vi "Set Message.vi"(8 "error in (no error)":errorcluster caption="entrée d'erreur (pas d'erreur)", 9 "Message type":T1="Control", 10 "Message.lvclass":refnum<class "Message.lvclass">, 11 "GeneralFunctionality en entrée":refnum<class "GeneralFunctionality.lvclass">) -> (0 "error out":errorcluster caption="sortie d'erreur", 3 "GeneralFunctionality en sortie":refnum<class "GeneralFunctionality.lvclass">)   [LabVIEW 2018, in "GeneralFunctionality.lvclass"]
uses:
  GeneralFunctionality.lvclass
  dependecies/ControlsVIs/Clusters-def/Message types.ctl
  Message/Message.lvclass
  GeneralFunctionality.lvclass/GeneralFunctionality.ctl
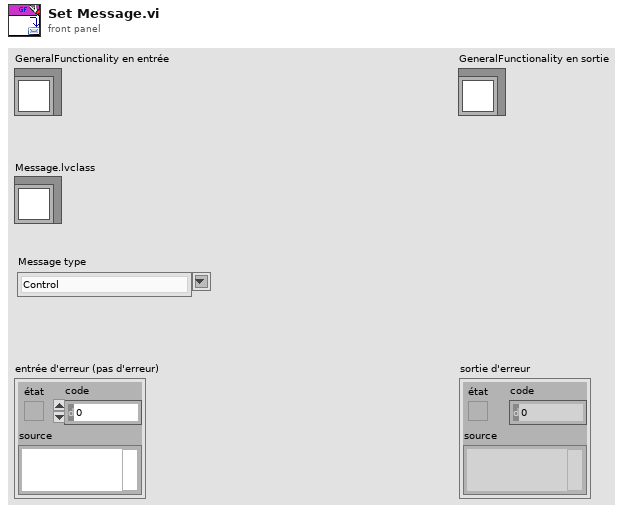
[diagram p1: front panel]
types:
  T1 = typedef "Message types.ctl" = string
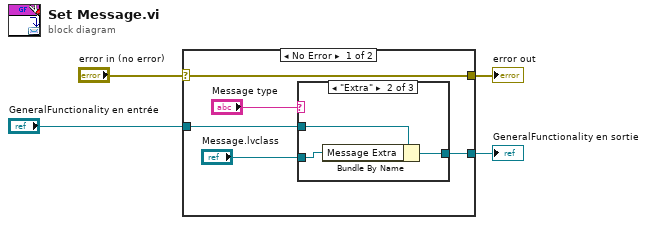
[diagram p0: block diagram]
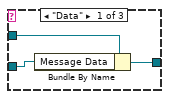
[diagram p2: hidden frame]
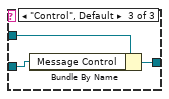
[diagram p3: hidden frame]
diagram:
  n1 = case shown="No Error" "error in (no error)" {
    selector: "error in (no error)" -> [w9 w20]
    tunnel: [w9 w20] -> w3
    tunnel: [w5 w19] -> w1
    tunnel: "GeneralFunctionality en entrée" -> [w6 w19]
    frame No Error {
      n2 = case shown="\"Extra\"" "Message type" {
        tunnel: w6 -> [w12 w15 w18]
        tunnel: [w10 w13 w17] -> w5
        tunnel: "Message.lvclass" -> [w11 w14 w16]
        frame "Data" {
          n3 = Bundle By Name(cluster=w12, "Message Data"=w11) -> (w10:refnum<class "GeneralFunctionality.lvclass">)
        }
        frame "Extra" {
          n4 = Bundle By Name(cluster=w15, "Message Extra"=w14) -> (w13:refnum<class "GeneralFunctionality.lvclass">)
        }
        frame "Control", Default {
          n5 = Bundle By Name(cluster=w18, "Message Control"=w16) -> (w17:refnum<class "GeneralFunctionality.lvclass">)
        }
      }
    }
    frame Error {
    }
  }
  "error out" <- w3
  "GeneralFunctionality en sortie" <- w1
